vi "RC_Test.vi"() -> ()   [LabVIEW 2013]
uses:
  <vilib>/rvi/interface/nirviOpenFPGA/nirviOpenFPGA.xnode
  Data/TypeDefs/DynamixelCycleTracker.ctl
  <instrlib>/Dynamixel Motor/Dynamixel Motor.lvlib
  FPGA Bitfiles/AutonomousSailbo_FPGATarget_myRIOPWMDecoder_uSRMj+uIEmA.lvbitx
  FPGA_Code/myRIO_PWM_Decoder.vi
  <vilib>/FPGAPlugInAG/myRIO-1900/niLvFpga_Open_myRIO-1900.vi
  <vilib>/rvi/interface/common/dynamic/niFpgaDynamicAddResources.vi
  Data/TypeDefs/Rudder Set Suggestions.ctl
panel:
  in  "Motors Enabled":bool[](array[boolean])=[TRUE, TRUE, TRUE]
  out "error out":errorcluster[](array[cluster])
  out "Motors IDs Found":u8[](array[numeric])
  out "Commanded rudder value":T1 min=-0.95 max=0.95 scale=1.0..-1.0
  out "Commanded sail value":dbl
  out "Write loop counter":i32
  out "Updated Dynamixel Cycles":T2
  out "Dynamixel Positions (deg)":dbl[](array[numeric])
  out "Read loop counter":i32
  in  "Stop reading":bool
  in  "Stop writing":bool
  in  "VISA resource name":refnum<visa-resource-name>="ASRL3::INSTR"
  # "Read from RC Controller"
  # "Read from Dynamixels"
  # "Check value rudder is being commanded to in position control"
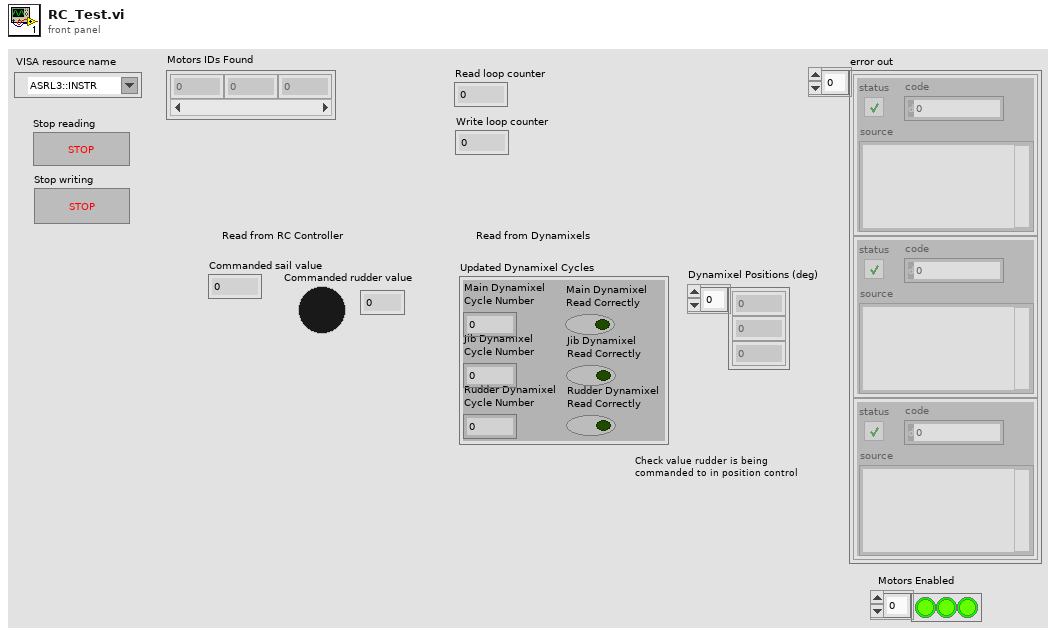
[diagram p1: front panel]
types:
  T1 = typedef "Rudder Set Suggestions.ctl" = dbl
  T2 = typedef "DynamixelCycleTracker.ctl" = cluster{"Main Dynamixel\nCycle Number":i32, "Jib Dynamixel\nCycle Number":i32, "Rudder Dynamixel\nCycle Number":i32, "Main Dynamixel\nRead Correctly":bool, "Jib Dynamixel\nRead Correctly":bool, "Rudder Dynamixel\nRead Correctly":bool}
  T3 = typedef "MotorSetup.ctl" = cluster{"Main Dynamixel Set Data":T4, "Rudder Dynamixel Set Data":T4, "Jib Dynamixel Set Data":T4}
  T4 = typedef "DynamixelSetupInfo.ctl" = cluster{"Lower Winch Bound (deg)":dbl, "Upper Winch Bound (deg)":dbl}
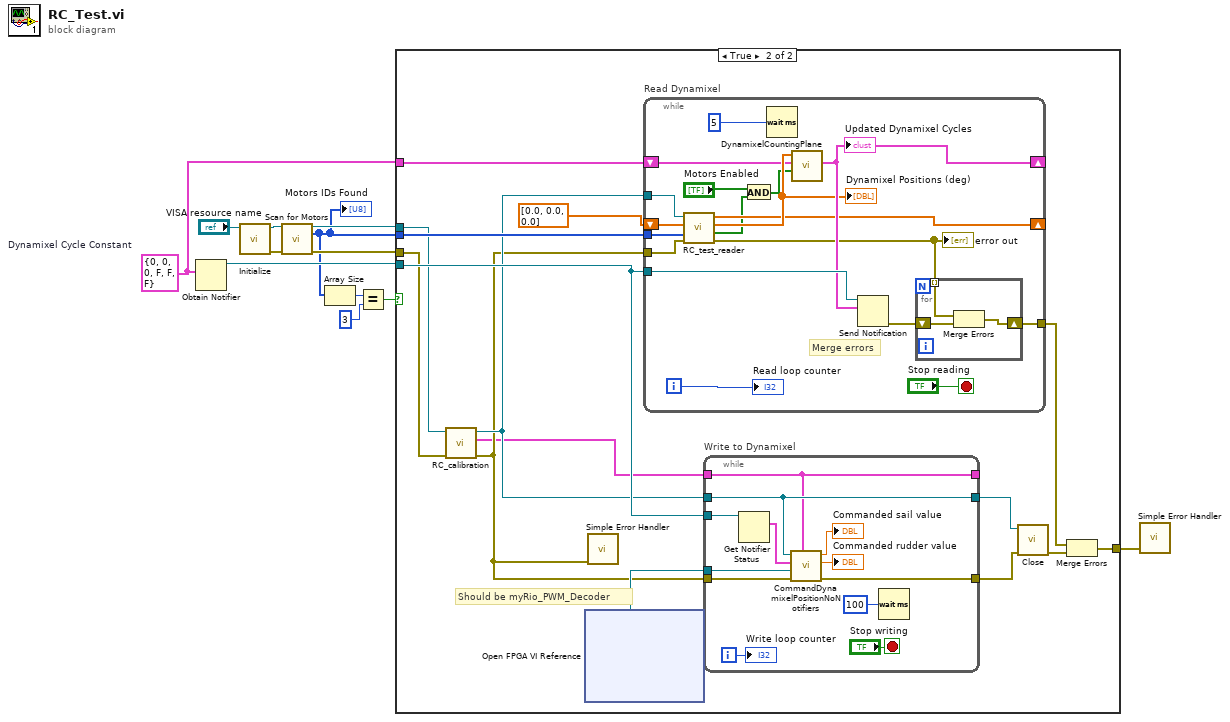
[diagram p0: block diagram]
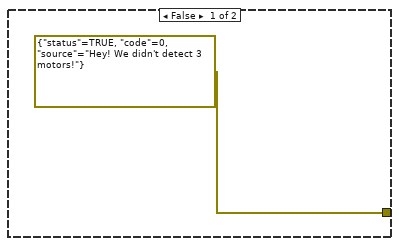
[diagram p2: hidden frame]
diagram:
  w8 = T2 {"Main Dynamixel\nCycle Number"=0, "Jib Dynamixel\nCycle Number"=0, "Rudder Dynamixel\nCycle Number"=0, "Main Dynamixel\nRead Correctly"=FALSE, "Jib Dynamixel\nRead Correctly"=FALSE, "Rudder Dynamixel\nRead Correctly"=FALSE}  # Dynamixel Cycle Constant
  n1 = Obtain Notifier(notification data type=w8) -> (notifier out=w12:refnum<notifier>)  [unwired: 3 in, 2 out]
  n2 = call <instrlib>:"Initialize.vi"("VISA resource name"="VISA resource name") -> ("error out"=w10:errorcluster, "VISA resource name out"=w9:refnum<visa-resource-name>)  [unwired: 9 in]
  n3 = call <instrlib>:"Scan for Motors.vi"("VISA resource name"=w9, "error in (no error)"=w10) -> ("VISA resource name out"=w7:refnum<visa-resource-name>, "Motors IDs Found"=w1:u8[], "error out"=w6:errorcluster)  [unwired: 11 in]
  "Motors IDs Found" <- w1
  n4 = Array Size(array=w1) -> (size(s)=w5:i32)
  n5 = Equal?(x=w5, y=3) -> (x = y?=w4:bool)
  n6 = case shown="True" w4 {
    tunnel: w12 -> [_ w20]
    tunnel: w8 -> [_ w27]
    tunnel: w1 -> [_ w26]
    tunnel: w7 -> [_ w18]
    tunnel: w6 -> [_ w17]
    tunnel: [errorcluster {"status"=TRUE, "code"=0, "source"="Hey! We didn't detect 3 motors!"} ("error IO") w23] -> w2
    frame False {
    }
    frame True {
      # "Should be myRio_PWM_Decoder"
      n7 = call "RC_calibration.vi"("error in (no error)"=w17, "VISA resource name"=w18) -> ("error IO"=w15:errorcluster, "Dynamixel Bounds Out"=w14:T3, "VISA resource name out"=w16:refnum<visa-resource-name>)  [unwired: 7 in]
      n8 = xnode "Open FPGA VI Reference"() -> ("FPGA VI Reference Out"=w28:refnum<k20>)  [unwired: 2 in, 1 out]
      n9 = call <vilib>:"Simple Error Handler.vi"("error in (no error)"=w15) -> ()  [unwired: 4 in, 5 out]
      n10 = while "Read Dynamixel" {
        tunnel: w16 -> [w57]
        shift-right: [w55] -> _
        shift-left: w27 -> [w47]
        tunnel: w20 -> [w56]
        tunnel: w26 -> [w53]
        tunnel: w15 -> [w58]
        shift-right: [w49] -> _
        shift-left: dbl[] [0.0, 0.0, 0.0] -> [w48]
        tunnel: [w44] -> w19
        i -> [w52]
        stop <- "Stop reading" stop-if-true
        # "Merge errors"
        n11 = call "RC_test_reader.vi"("error in (no error)"=w58, "Motors IDs Found"=w53, "Read positions (dyn)"=w48, "VISA Refnum in"=w57) -> ("error out"=w45:errorcluster[], "Motors Read Correctly"=w42:bool[], "Dynamixel Positions (deg)"=w51:dbl[], "Read positions latest (dyn)"=w49:dbl[])  [unwired: 3 in, 1 out]
        "Dynamixel Positions (deg)" <- w51
        "error out" <- w45
        n12 = And(x="Motors Enabled", y=w42) -> (x .and. y?=w43:bool[])
        n13 = Wait (ms)(milliseconds to wait=u32 5) -> ()  [unwired: 1 out]
        n14 = call "DynamixelCountingPlane.vi"("Motors Read Correctly"=w43, "Dynamixel Cycles"=w47, "Dynamixel Read Positions"=w51) -> ("Updated Dynamixle Cycles"=w55:T2)  [unwired: 8 in]
        "Updated Dynamixel Cycles" <- w55
        n15 = Send Notification(notification=w55, notifier=w56) -> (error out=w46:errorcluster)  [unwired: 1 in, 1 out]
        n16 = for {
          shift-right: [w61] -> w44
          shift-left: w46 -> [w60]
          tunnel: w45 -> [w59] mode=indexing
          n17 = Merge Errors(w59, w60) -> (w61:errorcluster)
        }
        "Read loop counter" <- w52
      }
      n18 = while "Write to Dynamixel" {
        tunnel: w28 -> [w40]
        tunnel: w16 -> [w33]
        tunnel: w20 -> [w39]
        tunnel: w15 -> [w37]
        tunnel: [w36] -> w21
        tunnel: [w33] -> w22
        tunnel: [w29] -> _
        tunnel: w14 -> [w29]
        i -> [w32]
        stop <- "Stop writing" stop-if-true
        n19 = Get Notifier Status(notifier=w39) -> (current notification=w38:T2)  [unwired: 1 in, 4 out]
        n20 = call "CommandDynamixelPositionNoNotifiers.vi"("Dynamixel Bounds"=w29, "error in"=w37, "FPGA VI Reference In"=w40, "Dynamixel Cycles"=w38, "VISA resource name"=w33) -> ("Error out"=w36:errorcluster, "Commanded rudder value"=→"Commanded rudder value":T1, "Debug sail value"=→"Commanded sail value":dbl)  [unwired: 3 in, 1 out]
        n21 = Wait (ms)(milliseconds to wait=u32 100) -> ()  [unwired: 1 out]
        "Write loop counter" <- w32
      }
      n22 = call <instrlib>:"Close.vi"("error in (no error)"=w21, "VISA resource name"=w22) -> ("error out"=w25:errorcluster)  [unwired: 9 in]
      n23 = Merge Errors(w19, w25) -> (w23:errorcluster)
    }
  }
  n24 = call <vilib>:"Simple Error Handler.vi"("error in (no error)"=w2) -> ()  [unwired: 4 in, 5 out]
